vi "SE5082_Load_waveform.vi"(8 "error in":errorcluster, 9 "Channel":u16(ring)=1 items=["Channel 1", "Channel 2"], 10 "waveform":dbl[](array[numeric])=array[97504 elements], 11 "VISA resource name in":refnum<visa-resource-name>="USB0::0x168C::0x5082::0000217419::INSTR") -> (0 "error out":errorcluster, 3 "VISA resource name out":refnum<visa-resource-name>="USB0::0x168C::0x5082::0000217419::INSTR")   [LabVIEW 2017]
panel:
  out "length":i32=195008
  out "Interlacing array":u8[](array[numeric])
  out "first 8 bits":u8[](array[numeric])
  out "last 8 bits":u8[](array[numeric])
  out "unsigned 16bit integer":u16[](array[numeric])
  in  "Readout status?":bool
  in  "Read-out commands":string[](array[string])=[":INST 1;:VOLT?", ":INST 1;:VOLT:OFFS?", ":INST 1;:OUTP?", ":INST 2;:VOLT?", ":INST 2;:VOLT:OFFS?", ":INST 2;:OUTP?"]
  out "Input waveform commands":string[](array[string])
  out "Status output":string[](array[string])=["1.000e+00\n", "0.000e+00\n", "ON\n", "5.000e-01\n", "0.000e+00\n", "ON\n"]
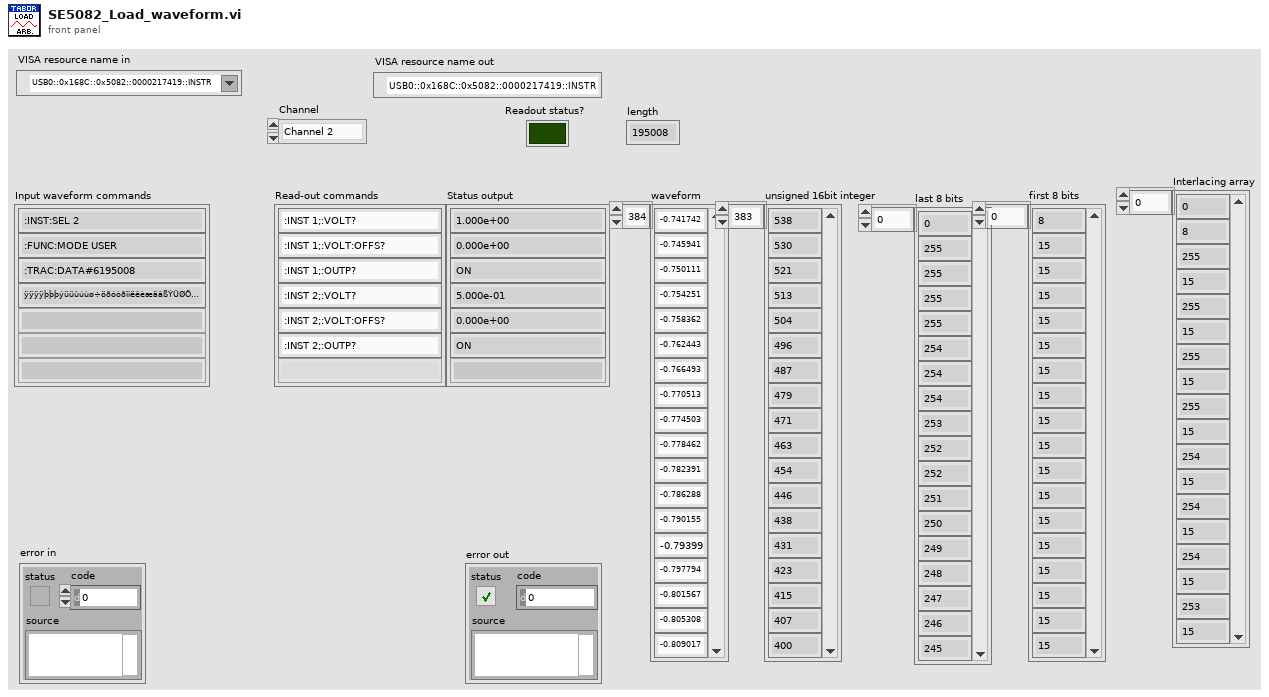
[diagram p1: front panel]
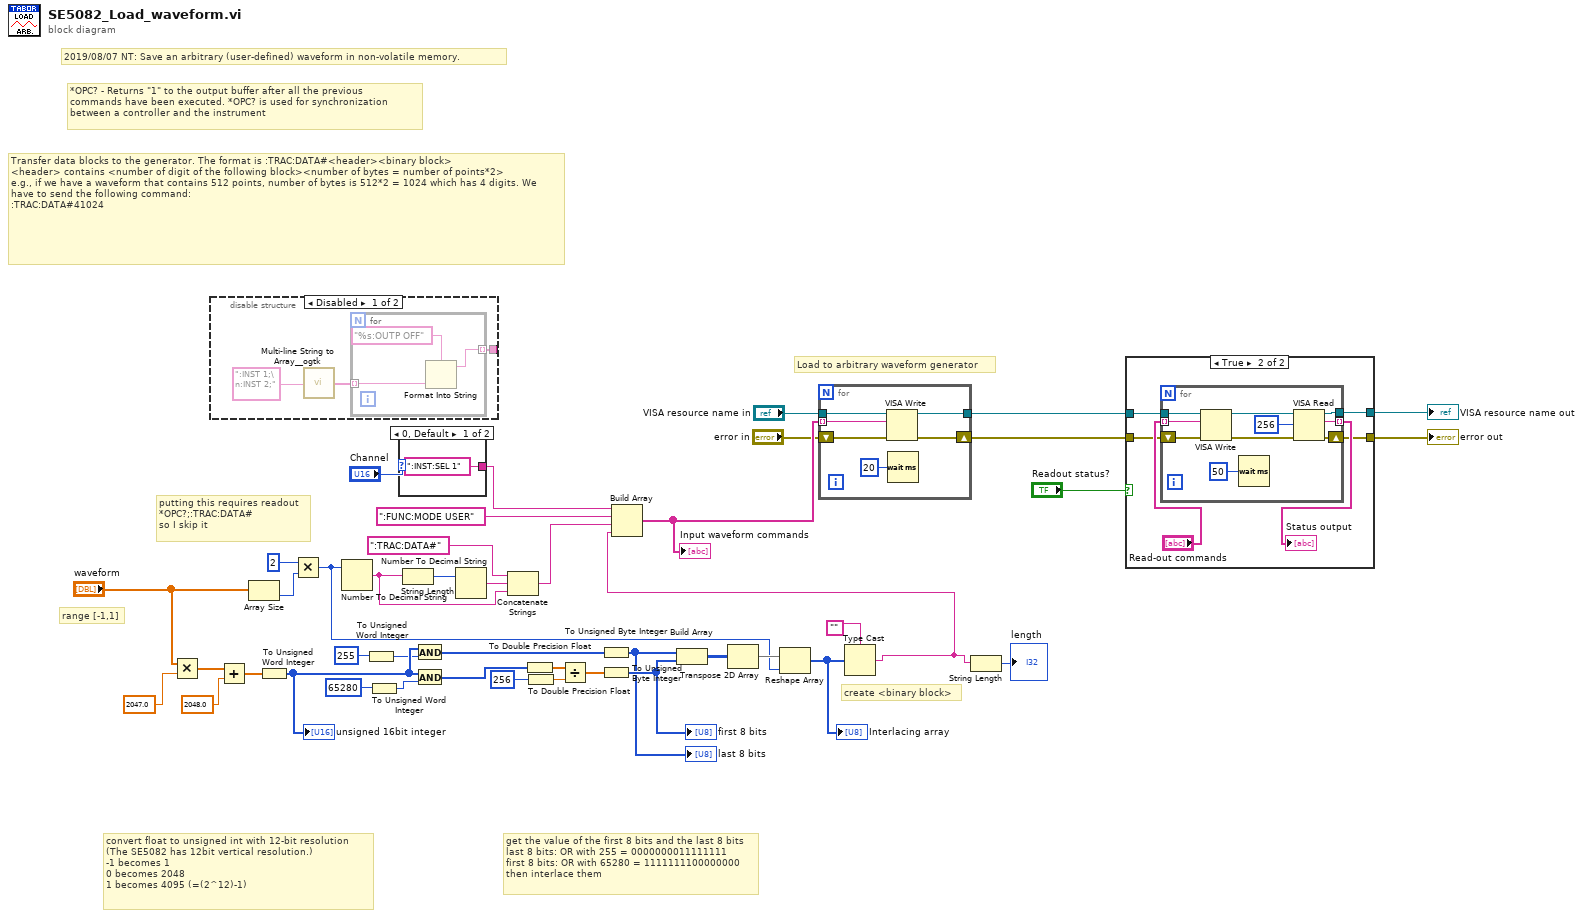
[diagram p0: block diagram]
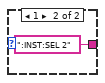
[diagram p3: hidden frame]
diagram:
  # "putting this requires readout\n*OPC?;:TRAC:DATA#\nso I skip it"
  # "create <binary block>"
  # "get the value of the first 8 bits and the last 8 bits\nlast 8 bits: OR with 255 = 0000000011111111 \nfirst 8 bits: OR with 65280 = 1111111100000000\nthen interlace them"
  # "convert float to unsigned int with 12-bit resolution\n(The SE5082 has 12bit vertical resolution.)\n-1 becomes 1\n0 becomes 2048\n1 becomes 4095 (=(2^12)-1)"
  # "range [-1,1]"
  # "*OPC? - Returns \"1\" to the output buffer after all the previous\ncommands have been executed. *OPC? is used for synchronization\nbetween a controller and the instrument"
  # "Transfer data blocks to the generator. The format is :TRAC:DATA#<header><binary block>\n<header> contains <number of digit of the following block><number of bytes = number of points*2> \ne.g., if we have a waveform that contains 512 points, number of bytes is 512*2 = 1024 which has 4 digits. We have to send the following command:\n:TRAC:DATA#41024"
  # "2019/08/07 NT: Save an arbitrary (user-defined) waveform in non-volatile memory."
  # "Load to arbitrary waveform generator"
  n1 = Multiply(x="waveform", y=2047.0) -> (x*y=w34:dbl[])
  n2 = disable-structure shown="Disabled" {
    disable-tunnel: [w44 _] -> _
    frame Disabled {
      n3 = call <userlib>:"Multi-line String to Array__ogtk.vi"("string"=":INST 1;\n:INST 2;" ("initial string")) -> ("lines"=w45:string[])
      n4 = for {
        tunnel: w45 -> [w47] mode=indexing
        tunnel: [w48] -> w44 mode=indexing
        n5 = Format Into String(format string="%s:OUTP OFF", w47) -> (resulting string=w48:string)  [unwired: 2 in, 1 out]
      }
    }
    frame Enabled {
    }
  }
  n6 = Add(x=w34, y=2048.0) -> (x+y=w35:dbl[])
  n7 = Array Size(array="waveform") -> (size(s)=w28:i32)
  n8 = To Unsigned Word Integer(number=w35) -> (unsigned 16bit integer=w32:u16[])
  "unsigned 16bit integer" <- w32
  n9 = Multiply(x=2, y=w28) -> (x*y=w16:i32)
  n10 = Number To Decimal String(number=w16) -> (decimal integer string=w17:string)  [unwired: 1 in]
  n11 = To Unsigned Word Integer(number=255) -> (unsigned 16bit integer=w29:u16)
  n12 = To Unsigned Word Integer(number=65280) -> (unsigned 16bit integer=w31:u16)
  n13 = case shown="0, Default" "Channel" {
    tunnel: [":INST:SEL 1" ("initial string") ":INST:SEL 2" ("initial string")] -> w10
    frame 0, Default {
    }
    frame 1 {
    }
  }
  n14 = String Length(string=w17) -> (length=w25:i32)
  n15 = And(x=w32, y=w29) -> (x .and. y?=w30:u16[])
  n16 = And(x=w32, y=w31) -> (x .and. y?=w15:u16[])
  n17 = Number To Decimal String(number=w25) -> (decimal integer string=w24:string)  [unwired: 1 in]
  n18 = Concatenate Strings(":TRAC:DATA#", w24, w17) -> (w41:string)
  n19 = To Double Precision Float(number=w15) -> (double precision float=w20:dbl[])
  n20 = To Double Precision Float(number=256) -> (double precision float=w18:dbl)
  n21 = Divide(x=w20, y=w18) -> (x/y=w33:dbl[])
  n22 = To Unsigned Byte Integer(number=w30) -> (unsigned 8bit integer=w12:u8[])
  "last 8 bits" <- w12
  n23 = To Unsigned Byte Integer(number=w33) -> (unsigned 8bit integer=w13:u8[])
  "first 8 bits" <- w13
  n24 = Build Array(w12, w13) -> (w23:u8[][])
  n25 = Transpose 2D Array(2D array=w23) -> (transposed array=w22:u8[][])
  n26 = Reshape Array(w22, w16) -> (w14:u8[])
  "Interlacing array" <- w14
  n27 = Type Cast(type="", x=w14) -> (*(type *) &x=w7:string)
  n28 = Build Array(w10, ":FUNC:MODE USER" ("write buffer"), w41, w7) -> (w9:string[])
  "Input waveform commands" <- w9
  n29 = for {
    tunnel: "VISA resource name in" -> [w57]
    tunnel: w9 -> [w56] mode=indexing
    shift-right: [w54] -> w5
    shift-left: "error in" -> [w55]
    tunnel: [w53] -> w6
    n30 = VISA Write(VISA resource name=w57, write buffer=w56, error in (no error)=w55) -> (VISA resource name out=w53:refnum<visa-resource-name>, error out=w54:errorcluster)  [unwired: 1 out]
    n31 = Wait (ms)(milliseconds to wait=u32 20) -> ()  [unwired: 1 out]
  }
  n32 = String Length(string=w7) -> (length=→"length":i32)
  n33 = case shown="True" "Readout status?" {
    tunnel: w6 -> [w59 w63]
    tunnel: w5 -> [w58 w62]
    tunnel: [w58 w61] -> w2
    tunnel: [w59 w60] -> w1
    frame False {
    }
    frame True {
      n34 = for {
        tunnel: [w72] -> w65 mode=indexing
        shift-right: [w71] -> w61
        shift-left: w62 -> [w68]
        tunnel: w63 -> [w70]
        tunnel: "Read-out commands" -> [w69] mode=indexing
        tunnel: [w66] -> w60
        n35 = VISA Write(VISA resource name=w70, write buffer=w69, error in (no error)=w68) -> (VISA resource name out=w74:refnum<visa-resource-name>, error out=w73:errorcluster)  [unwired: 1 out]
        n36 = Wait (ms)(milliseconds to wait=u32 50) -> ()  [unwired: 1 out]
        n37 = VISA Read(VISA resource name=w74, byte count=u32 256, error in (no error)=w73) -> (VISA resource name out=w66:refnum<visa-resource-name>, read buffer=w72:string, error out=w71:errorcluster)  [unwired: 1 out]
      }
      "Status output" <- w65
    }
  }
  "error out" <- w2
  "VISA resource name out" <- w1
